vi "PathFilterTest.vi"(11 "error in":errorcluster) -> (15 "error out":errorcluster)   [LabVIEW 2023, in "TestVIs.lvlib"]
uses:
  TestVIs.lvlib
  <vilib>/addons/_JKI Toolkits/Caraya/classes/Assert/Assert Equal Value_Variant.vi
  <vilib>/addons/_JKI Toolkits/Caraya/classes/Test/Test.lvclass
  Library/Unit Testing CA1.lvlib
  <vilib>/addons/_JKI Toolkits/Caraya/classes/Assert/Assert.lvclass
panel:
  # "PATH FILTER TEST"
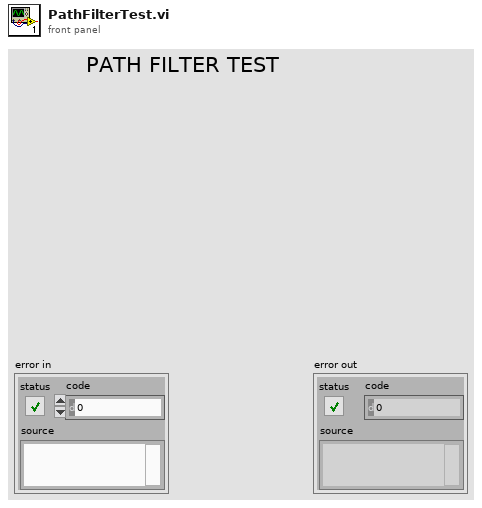
[diagram p1: front panel]
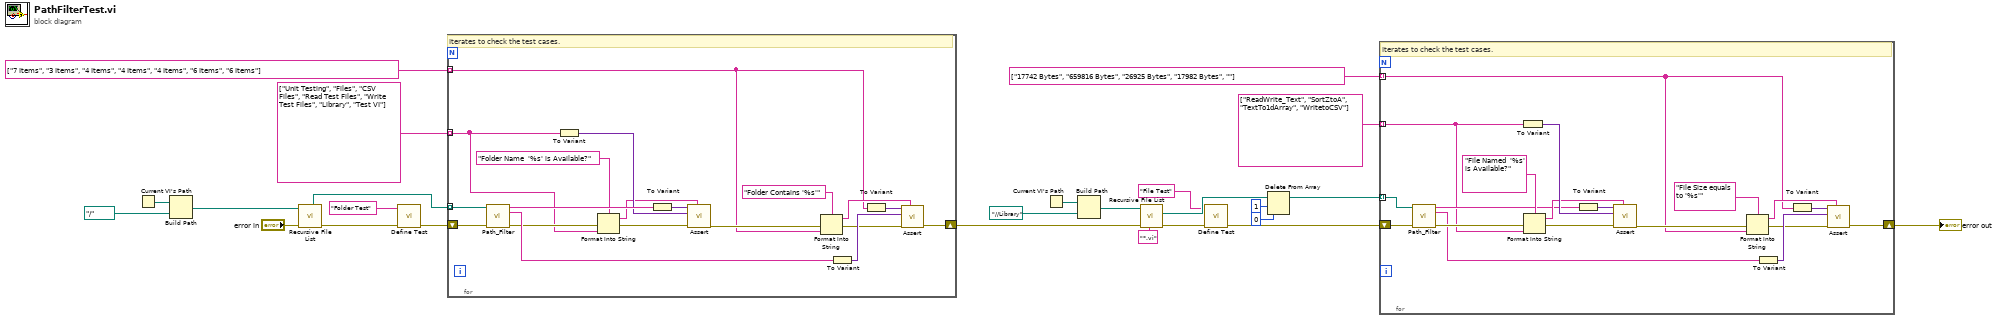
[diagram p0: block diagram]
diagram:
  n1 = Current VI's Path() -> (path=w12:path)
  n2 = Build Path(base path=w12, name or relative path=path "../..") -> (appended path=w9:path)
  n3 = call <vilib>:"Recursive File List.vi"("error in (no error)"="error in", "Folder Path"=w9) -> ("error out"=w10:errorcluster, "All Folders"=w8:path[])  [unwired: 5 in, 3 out]
  n4 = call <vilib>:"Define Test.vi"("error in (no error)"=w10, "Label (VI Title)"="Folder Test") -> ("error out"=w21:errorcluster)  [unwired: 8 in, 1 out]
  n5 = for {
    tunnel: w8 -> [w44] mode=indexing
    shift-right: [w38] -> w14
    shift-left: w21 -> [w43]
    tunnel: string[] ["Unit Testing", "Files", "CSV Files", "Read Test Files", "Write Test Files", "Library", "Test VI"] ("Array") -> [w27] mode=indexing
    tunnel: string[] ["7 Items", "3 Items", "4 Items", "4 Items", "4 Items", "6 Items", "6 Items"] ("Array 2") -> [w26] mode=indexing
    # "Iterates to check the test cases."
    n6 = call "Path_Filter.vi"("path"=w44, "error in"=w43) -> ("File/Folder Name"=w42:string, "Size"=w37:string, "error out"=w35:errorcluster)  [unwired: 11 in]
    n7 = To Variant(anything=w27) -> (Variant=w41:variant)
    n8 = Format Into String(format string="Folder Name  '%s' is Available?", error in=w35, w27) -> (resulting string=w32:string, error out=w34:errorcluster)  [unwired: 1 in]
    n9 = To Variant(anything=w42) -> (Variant=w40:variant)
    n10 = call-poly <vilib>:"Assert.vi"("Label"=w32, "error in (no error)"=w34, "Y"=w41, "X"=w40) -> ("error out"=w30:errorcluster)  [unwired: 6 in, 1 out]
    n11 = Format Into String(format string="Folder Contains '%s'", error in=w30, w26) -> (resulting string=w29:string, error out=w28:errorcluster)  [unwired: 1 in]
    n12 = To Variant(anything=w37) -> (Variant=w36:variant)
    n13 = To Variant(anything=w26) -> (Variant=w39:variant)
    n14 = call-poly <vilib>:"Assert.vi"("Label"=w29, "error in (no error)"=w28, "Y"=w36, "X"=w39) -> ("error out"=w38:errorcluster)  [unwired: 6 in, 1 out]
  }
  n15 = Current VI's Path() -> (path=w7:path)
  n16 = Build Path(base path=w7, name or relative path=path "../../Library") -> (appended path=w5:path)
  n17 = call <vilib>:"Recursive File List.vi"("pattern"="*.vi", "error in (no error)"=w14, "Folder Path"=w5) -> ("error out"=w17:errorcluster, "All Files in Dir"=w20:path[])  [unwired: 4 in, 3 out]
  n18 = call <vilib>:"Define Test.vi"("error in (no error)"=w17, "Label (VI Title)"="File Test") -> ("error out"=w16:errorcluster)  [unwired: 8 in, 1 out]
  n19 = Delete From Array(array=w20, length=1, index=0) -> (array with subset deleted=w3:path[])  [unwired: 1 out]
  n20 = for {
    tunnel: w3 -> [w63] mode=indexing
    shift-right: [w58] -> w13
    shift-left: w16 -> [w62]
    tunnel: string[] ["17742 Bytes", "659816 Bytes", "26925 Bytes", "17982 Bytes", ""] ("Array 2") -> [w45] mode=indexing
    tunnel: string[] ["ReadWrite_Text", "SortZtoA", "TextTo1dArray", "WritetoCSV"] ("Array") -> [w46] mode=indexing
    # "Iterates to check the test cases."
    n21 = call "Path_Filter.vi"("path"=w63, "error in"=w62) -> ("File/Folder Name"=w47:string, "Size"=w49:string, "error out"=w56:errorcluster)  [unwired: 11 in]
    n22 = To Variant(anything=w46) -> (Variant=w61:variant)
    n23 = Format Into String(format string="File Named  '%s' is Available?", error in=w56, w46) -> (resulting string=w53:string, error out=w55:errorcluster)  [unwired: 1 in]
    n24 = To Variant(anything=w47) -> (Variant=w60:variant)
    n25 = call-poly <vilib>:"Assert.vi"("Label"=w53, "error in (no error)"=w55, "Y"=w61, "X"=w60) -> ("error out"=w51:errorcluster)  [unwired: 6 in, 1 out]
    n26 = Format Into String(format string="File Size equals to '%s'", error in=w51, w45) -> (resulting string=w48:string, error out=w50:errorcluster)  [unwired: 1 in]
    n27 = To Variant(anything=w49) -> (Variant=w57:variant)
    n28 = To Variant(anything=w45) -> (Variant=w59:variant)
    n29 = call-poly <vilib>:"Assert.vi"("Label"=w48, "error in (no error)"=w50, "Y"=w57, "X"=w59) -> ("error out"=w58:errorcluster)  [unwired: 6 in, 1 out]
  }
  "error out" <- w13
